vi "SVFA Phase Unit Conversion.vi"   [LabVIEW 2017]
doc: "Converts phase spectra between degrees, radians, and cycles. Wire data to the <B>phase spectrum</B> input to determine the polymorphic instance to use or manually select the instance."
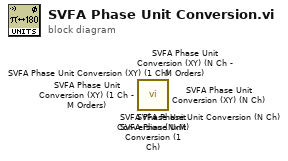
[diagram p0: block diagram]
diagram:
  n1 = call <vilib>:"SVFA Phase Unit Conversion (NxM).vi"() -> ()  [unwired: 16 in, 4 out]
  n2 = call <vilib>:"SVFA Phase Unit Conversion (XY) (N Ch - M Orders).vi"() -> ()  [unwired: 16 in, 4 out]
  n3 = call <vilib>:"SVFA Phase Unit Conversion (XY) (1 Ch - M Orders).vi"() -> ()  [unwired: 16 in, 4 out]
  n4 = call <vilib>:"SVFA Phase Unit Conversion (XY) (N Ch).vi"() -> ()  [unwired: 16 in, 4 out]
  n5 = call <vilib>:"SVFA Phase Unit Conversion (XY) (1 Ch).vi"() -> ()  [unwired: 16 in, 4 out]
  n6 = call <vilib>:"SVFA Phase Unit Conversion (N Ch).vi"() -> ()  [unwired: 16 in, 4 out]
  n7 = call <vilib>:"SVFA Phase Unit Conversion (1 Ch).vi"() -> ()  [unwired: 16 in, 4 out]
